vi "Engine-SystemAI-Channel.vi"(2 "Settings":T2, 3 "dt [s]":sgl=1.0 format="%0.2f", 4 "AI [V]":sgl) -> (0 "AI":sgl, 1 "AI":T3)   [LabVIEW 2016, in "DSI-RT.lvlib"]
uses:
  DSI-RT.lvlib
  Shared/Typedefs/Engine-Channel.ctl
  <vilib>/addons/Software Calibration Management/xSCM/Controls/TBL1D.ctl
  <vilib>/Analysis/3filter.llb/Filter Passband Type.ctl
  <vilib>/ptbypt/NI_PtbyPt.lvlib
  <vilib>/Analysis/NI_AALBase.lvlib
  Shared/DSI-Shared.lvlib
  <vilib>/addons/Software Calibration Management/xSCM/SCM-API.lvlib
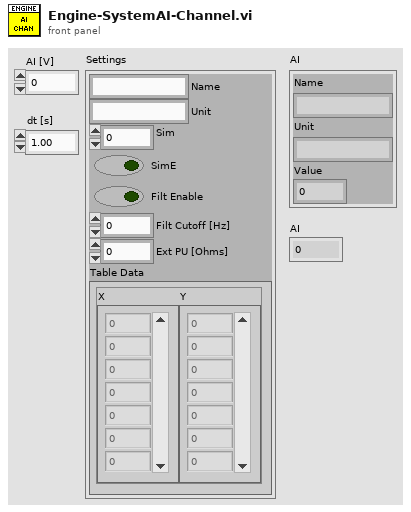
[diagram p1: front panel]
types:
  T1 = typedef "SCM-API.lvlib/TBL1D.ctl" = cluster{"X":sgl[], "Y":sgl[]}
  T2 = cluster{"Name":string, "Unit":string, "Sim":sgl, "SimE":bool, "Filt Enable":bool, "Filt Cutoff [Hz]":sgl, "Ext PU [Ohms]":sgl, "Table Data":T1}
  T3 = typedef "DSI-Shared.lvlib/Engine-Channel.ctl" = cluster{"Name":string, "Unit":string, "Value":sgl}
  T4 = typedef "NI_AALBase.lvlib/Filter Passband Type.ctl" = enum32{"Lowpass", "Highpass", "Bandpass", "Bandstop"}
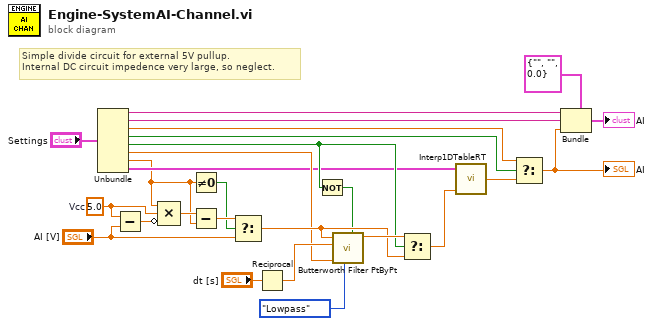
[diagram p0: block diagram]
diagram:
  w18 = sgl 5.0  # Vcc
  # "Simple divide circuit for external 5V pullup.  \nInternal DC circuit impedence very large, so neglect."
  n1 = Unbundle("Settings") -> ("Name"=w8:string, "Unit"=w7:string, "Sim"=w9:sgl, "SimE"=w10:bool, "Filt Enable"=w4:bool, "Filt Cutoff [Hz]"=w3:sgl, "Ext PU [Ohms]"=w1:sgl, "Table Data"=w2:T1)
  n2 = Subtract(x=w18, y="AI [V]") -> (x-y=w19:sgl)
  n3 = Compound Arithmetic op=MULTIPLY(w1, w18, invert w19) -> (w17:sgl)
  n4 = Not Equal To 0?(x=w1) -> (x != 0?=w15:bool)
  n5 = Subtract(x=w17, y=w1) -> (x-y=w16:sgl)
  n6 = Select(t=w16, s=w15, f="AI [V]") -> (s? t:f=w14:sgl)
  n7 = Reciprocal(x="dt [s]") -> (1/x=w25:sgl)
  n8 = Not(x=w4) -> (.not. x?=w11:bool)
  n9 = call <vilib>:"Butterworth Filter PtByPt.vi"("initialize"=w11, "filter type"=Filter_Passband_Type."Lowpass", "low cutoff freq: fl"=w3, "sampling freq: fs"=w25, "x"=w14) -> ("Filtered x"=w23:dbl)  [unwired: 4 in, 1 out]
  n10 = Select(t=w23, s=w4, f=w14) -> (s? t:f=w6:dbl)
  n11 = call <vilib>:"Interp1DTableRT.vi"("X"=w6, "1DTable"=w2) -> ("Y"=w5:sgl)  [unwired: 1 in]
  n12 = Select(t=w9, s=w10, f=w5) -> (s? t:f=w20:sgl)
  "AI" <- w20
  n13 = Bundle(cluster=T3 {"Name"="", "Unit"="", "Value"=0.0} ("AI01"), "Name"=w8, "Unit"=w7, "Value"=w20) -> (→"AI":T3)
